vi "Create FP Item.vi"(6 "Cluster Component":bool, 8 "error in (no error)":errorcluster, 10 "GObject In":refnum<vi>, 11 "GControl in":refnum<class "Control.lvclass">) -> (0 "error out":errorcluster, 1 "Is Control":bool, 2 "Is Indicator":bool, 3 "GControl out":refnum<class "Control.lvclass">, 4 "All Objects Created":refnum<class "Object.lvclass">[](array[class]), 5 "Is Visible":bool)   [LabVIEW 2017, in "Front Panel Publisher.lvlib" / "Control.lvclass"]
uses:
  Control.lvclass
  Text_class/Text.lvclass
  Text_class/Enum - Create Text Method.ctl
  Object_class/Object.lvclass
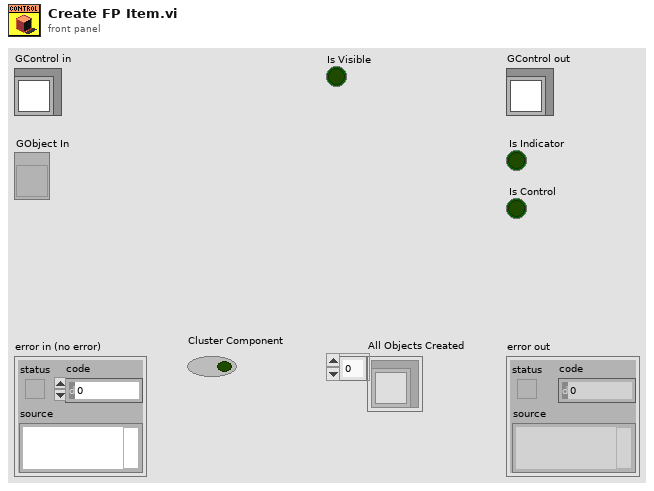
[diagram p1: front panel]
types:
  T1 = typedef "Front Panel Publisher.lvlib/Text.lvclass/Enum - Create Text Method.ctl" = enum16{"Text", "Label", "Caption", "Boolean Text"}
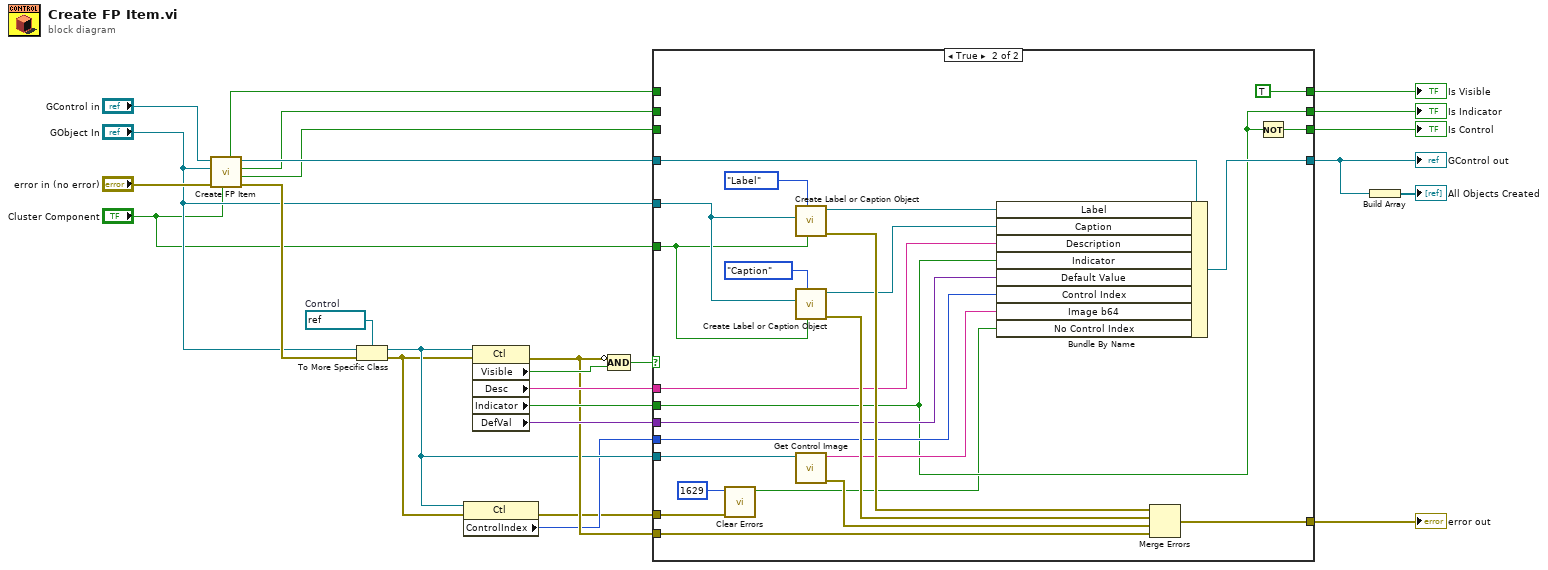
[diagram p0: block diagram]
diagram:
  w19 = refnum<vi> refnum  # Control
  n1 = call-parent "Create FP Item.vi"("Cluster Component"="Cluster Component", "error in (no error)"="error in (no error)", "GObject In"="GObject In", "GObject in"="GControl in") -> ("error out"=w18:errorcluster, "Is Control"=w11:bool, "Is Indicator"=w12:bool, "GObject out"=w14:refnum<class "Control.lvclass">, "Is Visible"=w13:bool)  [unwired: 2 in, 1 out]
  n2 = To More Specific Class(target class=w19, reference="GObject In", error in=w18) -> (specific class reference=w7:refnum<vi>, error out=w6:errorcluster)
  n3 = property class="Ctl"(reference=w7, error in=w6) -> (error out=w4:errorcluster, "ControlIndex"=w5:i32)  [unwired: 1 out]
  n4 = property class="Ctl"(reference=w7, error in=w6) -> (error out=w16:errorcluster, "Visible"=w20:bool, "Desc"=w24:string, "Indicator"=w23:bool, "DefVal"=w22:variant)  [unwired: 1 out]
  n5 = Compound Arithmetic op=AND(invert w16, w20) -> (w21:bool)
  n6 = case shown="True" w21 {
    tunnel: w24 -> [_ w44]
    tunnel: w23 -> [_ w39]
    tunnel: w22 -> [_ w43]
    tunnel: w5 -> [_ w42]
    tunnel: w7 -> [_ w55]
    tunnel: "GObject In" -> [_ w54]
    tunnel: w16 -> [w31 w50]
    tunnel: [w31 w49] -> w15
    tunnel: w14 -> [w30 w48]
    tunnel: [w30 w47] -> w3
    tunnel: w13 -> [w29 _]
    tunnel: w12 -> [w28 _]
    tunnel: w11 -> [w27 _]
    tunnel: [w29 TRUE ("Is Visible")] -> w10
    tunnel: [w28 w39] -> w9
    tunnel: [w27 w38] -> w8
    tunnel: w4 -> [_ w34]
    tunnel: "Cluster Component" -> [_ w32]
    frame False {
    }
    frame True {
      n7 = call <vilib>:"Clear Errors.vi"("error in (no error)"=w34, "specific error code to clear (0: all)"=1629) -> ("specific error cleared?"=w33:bool)  [unwired: 4 in, 1 out]
      n8 = call "Create Label or Caption Object.vi"("Cluster Component"=w32, "Text Type"=Enum_-_Create_Text_Method."Label", "GObject"=w54) -> ("error out"=w53:errorcluster, "Text out"=w46:refnum<class "Text.lvclass">)  [unwired: 7 in]
      n9 = call "Create Label or Caption Object.vi"("Cluster Component"=w32, "Text Type"=Enum_-_Create_Text_Method."Caption", "GObject"=w54) -> ("error out"=w52:errorcluster, "Text out"=w45:refnum<class "Text.lvclass">)  [unwired: 7 in]
      n10 = call "Get Control Image.vi"("Control ref"=w55) -> ("error out"=w51:errorcluster, "base64 encoded <img>"=w41:string)  [unwired: 8 in, 1 out]
      n11 = Bundle By Name(cluster=w48, "Label"=w46, "Caption"=w45, "Description"=w44, "Indicator"=w39, "Default Value"=w43, "Control Index"=w42, "Image b64"=w41, "No Control Index"=w33) -> (w47:refnum<class "Control.lvclass">)
      n12 = Merge Errors(w53, w52, w51, w50) -> (w49:errorcluster)
      n13 = Not(x=w39) -> (.not. x?=w38:bool)
    }
  }
  "error out" <- w15
  "GControl out" <- w3
  "Is Indicator" <- w9
  "Is Control" <- w8
  "Is Visible" <- w10
  n14 = Build Array(w3) -> (→"All Objects Created":refnum<class "Control.lvclass">[])
